vi "Read Port.vi"(8 "error in (no error)":errorcluster, 9 "Port 2":u16, 10 "VISA resource name":refnum<visa-resource-name>, 11 "Serial Device in":refnum<class "Serial Device.lvclass">) -> (0 "error out":errorcluster, 1 "Array":bool[](array[boolean]), 2 "VISA resource name 2":refnum<visa-resource-name>, 3 "Serial Device out":refnum<class "Serial Device.lvclass">)   [LabVIEW 2020, in "Serial Device.lvclass"]
uses:
  Serial Device.lvclass
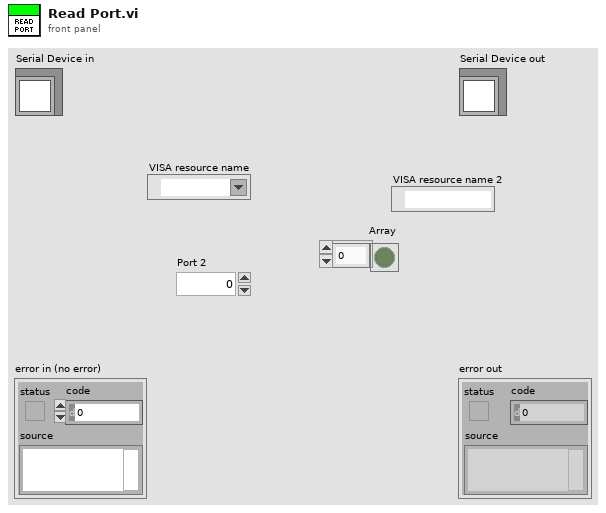
[diagram p1: front panel]
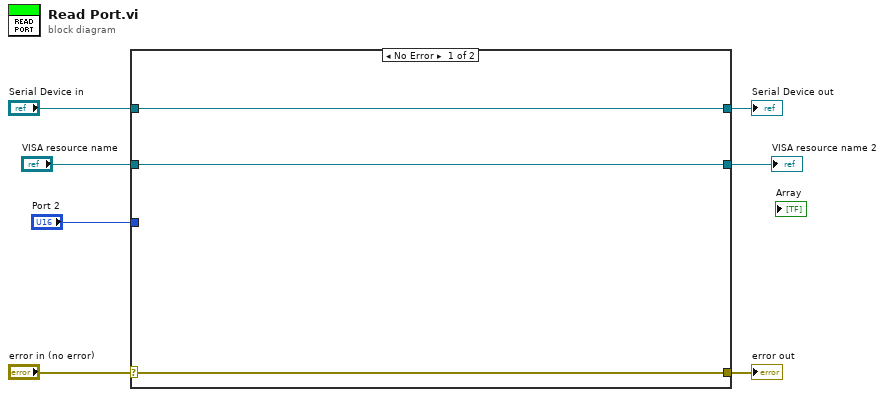
[diagram p0: block diagram]
diagram:
  n1 = case shown="No Error" "error in (no error)" {
    selector: "error in (no error)" -> [w9 w13]
    tunnel: [w9 w13] -> w6
    tunnel: [w10 w12] -> w4
    tunnel: "Serial Device in" -> [w10 w12]
    tunnel: "VISA resource name" -> [w8 w11]
    tunnel: "Port 2" -> [_ _]
    tunnel: [w8 w11] -> w1
    frame No Error {
    }
    frame Error {
    }
  }
  "error out" <- w6
  "Serial Device out" <- w4
  "VISA resource name 2" <- w1
